vi "openDevices.vi"(7 "Record Period":u16(ring)=9 items=["1 Millisecond", "2 Milliseconds", "5 Milliseconds", "10 Milliseconds", "20 Milliseconds", "50 Milliseconds", "100 Milliseconds", "200 Milliseconds", "500 Milliseconds", "1 Second", "2 Seconds", "5 Seconds", "10 Seconds", "20 Seconds", "1 Minute", "2 Minutes", "5 Minutes", "10 Minutes", "20 Minutes"], 8 "Chemin de sortie":path, 9 "Nom de l'analyse":string, 10 "Nom VISA d'entrée":refnum<visa-resource-name>, 11 "Numéro de série (PSI - 9200)":string) -> (0 "Das trouvé/configuré":bool, 1 "Erreur de sortie":errorcluster, 2 "Acq ID de sortie":T1, 3 "PSI_ID":string[](array[string]), 4 "Alim connectée":bool, 5 "Machines trouvées":string[][](array[string]), 6 "Numéro de la\nprochaine analyse":i32)   [LabVIEW 2019]
doc: "Il va ouvrer les connections avec le DAS240 et le EA-PSI 9200-25. Pour le premier, il sera sélectionné avec l'adresse IP de la machine voulue autant que l'alim est sélectionné avec le numéro de série."
uses:
  <instrlib>/Sefram DAS240/Public/Configure/Channels/Low-level/Set Type Voltage.vi
  <instrlib>/Sefram DAS240/Sefram DAS240.lvlib
panel:
  out "chaîne concaténée":string
  # "Les deux doit être vert"
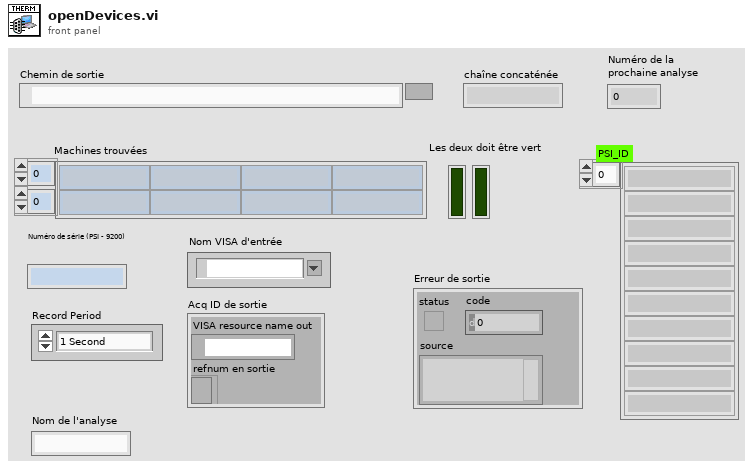
[diagram p1: front panel]
types:
  T1 = cluster{"VISA resource name out":refnum<visa-resource-name>, "refnum en sortie":refnum<file>}
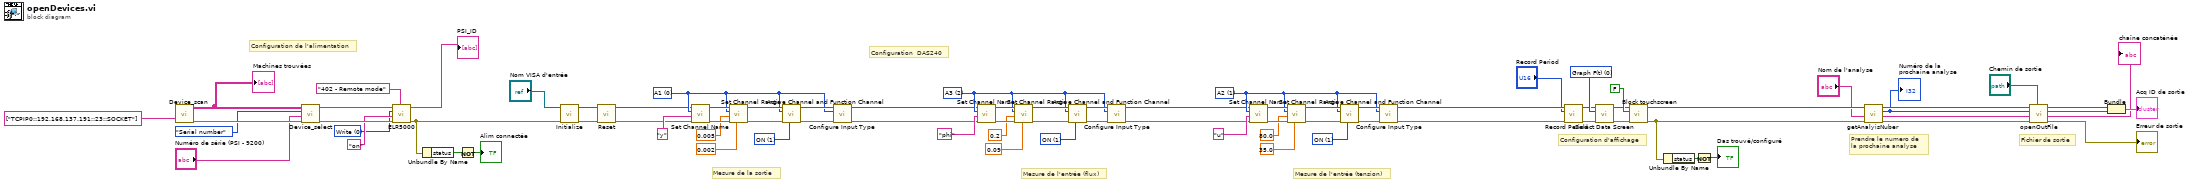
[diagram p0: block diagram]
diagram:
  w15 = u16 1 items=["OFF", "ON"] ("Channel State")
  w12 = u16 2 items=["A1", "A2", "A3", "A4", "A5", "A6", "A7", "A8", "A9", "A10", "A11", "A12", "A13", "A14", "A15", "A16", "A17", "A18", "A19", "A20", "B1", "B2", "B3", "B4", "B5", "B6", "B7", "B8", "B9", "B10", "B11", "B12", "B13", "B14", "B15", "B16", "B17", "B18", "B19", "B20", "C1", "C2", "C3", "C4", "C5", "C6", "C7", "C8", "C9", "C10", "C11", "C12", "C13", "C14", "C15", "C16", "C17", "C18", "C19", "C20", "D1", "D2", "D3", "D4", "D5", "D6", "D7", "D8", "D9", "D10", "D11", "D12", "D13", "D14", "D15", "D16", "D17", "D18", "D19", "D20", "E1", "E2", "E3", "E4", "E5", "E6", "E7", "E8", "E9", "E10", "E11", "E12", "E13", "E14", "E15", "E16", "E17", "E18", "E19", "E20", "F1", "F2", "F3", "F4", "F5", "F6", "F7", "F8", "F9", "F10", "F11", "F12", "F13", "F14", "F15", "F16", "F17", "F18", "F19", "F20", "G1", "G2", "G3", "G4", "G5", "G6", "G7", "G8", "G9", "G10", "G11", "G12", "G13", "G14", "G15", "G16", "G17", "G18", "G19", "G20", "H1", "H2", "H3", "H4", "H5", "H6", "H7", "H8", "H9", "H10", "H11", "H12", "H13", "H14", "H15", "H16", "H17", "H18", "H19", "H20", "I1", "I2", "I3", "I4", "I5", "I6", "I7", "I8", "I9", "I10", "I11", "I12", "I13", "I14", "I15", "I16", "I17", "I18", "I19", "I20", "J1", "J2", "J3", "J4", "J5", "J6", "J7", "J8", "J9", "J10", "J11", "J12", "J13", "J14", "J15", "J16", "J17", "J18", "J19", "J20", "K1", "K2", "K3", "K4"] ("Channel")
  w33 = u16 0 items=["Graph F(t)", "Numeric (DMM)", "Graph XY"] ("Screen display")
  w45 = u8 0 items=["Write", "Read"] ("Access")
  w63 = u16 1 items=["OFF", "ON"] ("Channel State")
  w57 = u16 1 items=["A1", "A2", "A3", "A4", "A5", "A6", "A7", "A8", "A9", "A10", "A11", "A12", "A13", "A14", "A15", "A16", "A17", "A18", "A19", "A20", "B1", "B2", "B3", "B4", "B5", "B6", "B7", "B8", "B9", "B10", "B11", "B12", "B13", "B14", "B15", "B16", "B17", "B18", "B19", "B20", "C1", "C2", "C3", "C4", "C5", "C6", "C7", "C8", "C9", "C10", "C11", "C12", "C13", "C14", "C15", "C16", "C17", "C18", "C19", "C20", "D1", "D2", "D3", "D4", "D5", "D6", "D7", "D8", "D9", "D10", "D11", "D12", "D13", "D14", "D15", "D16", "D17", "D18", "D19", "D20", "E1", "E2", "E3", "E4", "E5", "E6", "E7", "E8", "E9", "E10", "E11", "E12", "E13", "E14", "E15", "E16", "E17", "E18", "E19", "E20", "F1", "F2", "F3", "F4", "F5", "F6", "F7", "F8", "F9", "F10", "F11", "F12", "F13", "F14", "F15", "F16", "F17", "F18", "F19", "F20", "G1", "G2", "G3", "G4", "G5", "G6", "G7", "G8", "G9", "G10", "G11", "G12", "G13", "G14", "G15", "G16", "G17", "G18", "G19", "G20", "H1", "H2", "H3", "H4", "H5", "H6", "H7", "H8", "H9", "H10", "H11", "H12", "H13", "H14", "H15", "H16", "H17", "H18", "H19", "H20", "I1", "I2", "I3", "I4", "I5", "I6", "I7", "I8", "I9", "I10", "I11", "I12", "I13", "I14", "I15", "I16", "I17", "I18", "I19", "I20", "J1", "J2", "J3", "J4", "J5", "J6", "J7", "J8", "J9", "J10", "J11", "J12", "J13", "J14", "J15", "J16", "J17", "J18", "J19", "J20", "K1", "K2", "K3", "K4"] ("Channel")
  w71 = u16 1 items=["OFF", "ON"] ("Channel State")
  w60 = u16 0 items=["A1", "A2", "A3", "A4", "A5", "A6", "A7", "A8", "A9", "A10", "A11", "A12", "A13", "A14", "A15", "A16", "A17", "A18", "A19", "A20", "B1", "B2", "B3", "B4", "B5", "B6", "B7", "B8", "B9", "B10", "B11", "B12", "B13", "B14", "B15", "B16", "B17", "B18", "B19", "B20", "C1", "C2", "C3", "C4", "C5", "C6", "C7", "C8", "C9", "C10", "C11", "C12", "C13", "C14", "C15", "C16", "C17", "C18", "C19", "C20", "D1", "D2", "D3", "D4", "D5", "D6", "D7", "D8", "D9", "D10", "D11", "D12", "D13", "D14", "D15", "D16", "D17", "D18", "D19", "D20", "E1", "E2", "E3", "E4", "E5", "E6", "E7", "E8", "E9", "E10", "E11", "E12", "E13", "E14", "E15", "E16", "E17", "E18", "E19", "E20", "F1", "F2", "F3", "F4", "F5", "F6", "F7", "F8", "F9", "F10", "F11", "F12", "F13", "F14", "F15", "F16", "F17", "F18", "F19", "F20", "G1", "G2", "G3", "G4", "G5", "G6", "G7", "G8", "G9", "G10", "G11", "G12", "G13", "G14", "G15", "G16", "G17", "G18", "G19", "G20", "H1", "H2", "H3", "H4", "H5", "H6", "H7", "H8", "H9", "H10", "H11", "H12", "H13", "H14", "H15", "H16", "H17", "H18", "H19", "H20", "I1", "I2", "I3", "I4", "I5", "I6", "I7", "I8", "I9", "I10", "I11", "I12", "I13", "I14", "I15", "I16", "I17", "I18", "I19", "I20", "J1", "J2", "J3", "J4", "J5", "J6", "J7", "J8", "J9", "J10", "J11", "J12", "J13", "J14", "J15", "J16", "J17", "J18", "J19", "J20", "K1", "K2", "K3", "K4"] ("Channel")
  # "Prendre le numero de \nla prochaine analyse"
  # "Mesure de l'entrée (flux)"
  # "Configuration d'affichage"
  # "Fichier de sortie"
  # "Mesure de la sortie"
  # "Mesure de l'entrée (tension)"
  # "Configuration de l'alimentation"
  # "Configuration  DAS240"
  n1 = call <instrlib>:"Device_scan.vi"("Ports to skip"=string[] ["TCPIP0::192.168.137.191::23::SOCKET"]) -> ("Device information array"=w54:string[][], "error out"=w53:errorcluster)  [unwired: 1 in, 2 out]
  "Machines trouvées" <- w54
  n2 = call <instrlib>:"Device_select.vi"("error in (no error)"=w53, "Alias"="Numéro de série (PSI - 9200)", "Open by"=enum16{"Device Node", "Serial number", "Port"}."Serial number", "Device information array"=w54) -> ("error out"=w51:errorcluster, "Device information"=w52:string[])  [unwired: 3 in]
  n3 = call <instrlib>:"ELR5000.vi"("Command list"="402 - Remote mode", "Error in"=w51, "Value"="on", "Access"=w45, "Device information in"=w52) -> ("Error out"=w42:errorcluster, "Device information out"=→"PSI_ID":string[])  [unwired: 1 in, 2 out]
  n4 = Unbundle By Name(w42) -> ("status"=w50:bool)
  n5 = Not(x=w50) -> (.not. x?=→"Alim connectée":bool)
  n6 = call <instrlib>:"Initialize.vi"("error in (no error)"=w42, "VISA resource name"="Nom VISA d'entrée") -> ("error out"=w26:errorcluster, "VISA resource name out"=w27:refnum<visa-resource-name>)  [unwired: 8 in]
  n7 = call <instrlib>:"Reset.vi"("error in (no error)"=w26, "VISA resource name"=w27) -> ("error out"=w24:errorcluster, "VISA resource name out"=w25:refnum<visa-resource-name>)  [unwired: 8 in]
  n8 = call <instrlib>:"Set Channel Name.vi"("error in (no error)"=w24, "Channel name"="y", "Channel"=w60, "VISA resource name"=w25) -> ("error out"=w76:errorcluster, "VISA resource name out"=w77:refnum<visa-resource-name>)  [unwired: 6 in]
  n9 = call <instrlib>:"Set Channel Range.vi"("Center (in actual channel unit)"=0.002, "error in (no error)"=w76, "Channel range (in actual channel unit)"=0.005, "Channel"=w60, "VISA resource name"=w77) -> ("error out"=w72:errorcluster, "VISA resource name out"=w73:refnum<visa-resource-name>)  [unwired: 5 in]
  n10 = call <instrlib>:"Active Channel and Function Channel.vi"("Channel State"=w71, "error in (no error)"=w72, "Channel"=w60, "VISA resource name"=w73) -> ("error out"=w61:errorcluster, "VISA resource name out"=w62:refnum<visa-resource-name>)  [unwired: 6 in]
  n11 = call-poly <instrlib>:"Configure Input Type.vi"("error in (no error)"=w61, "Channel"=w60, "VISA resource name"=w62) -> ("error out"=w10:errorcluster, "VISA resource name out"=w11:refnum<visa-resource-name>)  [unwired: 7 in]
  n12 = call <instrlib>:"Set Channel Name.vi"("error in (no error)"=w10, "Channel name"="phi", "Channel"=w12, "VISA resource name"=w11) -> ("error out"=w20:errorcluster, "VISA resource name out"=w21:refnum<visa-resource-name>)  [unwired: 6 in]
  n13 = call <instrlib>:"Set Channel Range.vi"("Center (in actual channel unit)"=0.09, "error in (no error)"=w20, "Channel range (in actual channel unit)"=0.2, "Channel"=w12, "VISA resource name"=w21) -> ("error out"=w16:errorcluster, "VISA resource name out"=w17:refnum<visa-resource-name>)  [unwired: 5 in]
  n14 = call <instrlib>:"Active Channel and Function Channel.vi"("Channel State"=w15, "error in (no error)"=w16, "Channel"=w12, "VISA resource name"=w17) -> ("error out"=w14:errorcluster, "VISA resource name out"=w13:refnum<visa-resource-name>)  [unwired: 6 in]
  n15 = call-poly <instrlib>:"Configure Input Type.vi"("error in (no error)"=w14, "Channel"=w12, "VISA resource name"=w13) -> ("error out"=w8:errorcluster, "VISA resource name out"=w9:refnum<visa-resource-name>)  [unwired: 7 in]
  n16 = call <instrlib>:"Set Channel Name.vi"("error in (no error)"=w8, "Channel name"="u", "Channel"=w57, "VISA resource name"=w9) -> ("error out"=w68:errorcluster, "VISA resource name out"=w69:refnum<visa-resource-name>)  [unwired: 6 in]
  n17 = call <instrlib>:"Set Channel Range.vi"("Center (in actual channel unit)"=35.0, "error in (no error)"=w68, "Channel range (in actual channel unit)"=80.0, "Channel"=w57, "VISA resource name"=w69) -> ("error out"=w64:errorcluster, "VISA resource name out"=w65:refnum<visa-resource-name>)  [unwired: 5 in]
  n18 = call <instrlib>:"Active Channel and Function Channel.vi"("Channel State"=w63, "error in (no error)"=w64, "Channel"=w57, "VISA resource name"=w65) -> ("error out"=w59:errorcluster, "VISA resource name out"=w58:refnum<visa-resource-name>)  [unwired: 6 in]
  n19 = call-poly <instrlib>:"Configure Input Type.vi"("error in (no error)"=w59, "Channel"=w57, "VISA resource name"=w58) -> ("error out"=w41:errorcluster, "VISA resource name out"=w40:refnum<visa-resource-name>)  [unwired: 7 in]
  n20 = call <instrlib>:"Record Period.vi"("error in (no error)"=w41, "Record Period"="Record Period", "VISA resource name"=w40) -> ("error out"=w31:errorcluster, "VISA resource name out"=w32:refnum<visa-resource-name>)  [unwired: 7 in]
  n21 = call <instrlib>:"Select Data Screen.vi"("error in (no error)"=w31, "Screen display"=w33, "VISA resource name"=w32) -> ("error out"=w30:errorcluster, "VISA resource name out"=w29:refnum<visa-resource-name>)  [unwired: 7 in]
  n22 = call <instrlib>:"Block touchscreen.vi"("error in (no error)"=w30, "Block touchscreen?"=FALSE, "VISA resource name"=w29) -> ("error out"=w7:errorcluster, "VISA resource name out"=w4:refnum<visa-resource-name>)  [unwired: 7 in]
  n23 = Unbundle By Name(w7) -> ("status"=w80:bool)
  n24 = Not(x=w80) -> (.not. x?=→"Das trouvé/configuré":bool)
  n25 = call "getAnalyisNuber.vi"("Erreur en entrée"=w7, "Nom de l'analyse en entrée"="Nom de l'analyse", "VISA resource en entrée"=w4) -> ("error out"=w6:errorcluster, "Nom de l'analyse en sortie"=w1:string, "Numéro de la\nprochaine analyse"=w3:i32, "VISA resource en sortie"=w5:refnum<visa-resource-name>)  [unwired: 5 in]
  "Numéro de la\nprochaine analyse" <- w3
  n26 = call "openOutFile.vi"("Chemin de sortie"="Chemin de sortie", "Entrée d'erreur"=w6, "Nom de l'analyse"=w1, "Num de l'analyse"=w3, "VISA resource name"=w5) -> ("Sortie d'erreur"=→"Erreur de sortie":errorcluster, "chaîne concaténée"=→"chaîne concaténée":string, "refnum en sortie"=w37:refnum<file>, "VISA resource name out"=w38:refnum<visa-resource-name>)  [unwired: 2 in, 1 out]
  n27 = Bundle("VISA resource name out"=w38, "refnum en sortie"=w37) -> (→"Acq ID de sortie":T1)  [unwired: 1 in]
